vi "Bildunterschrifft.vi"(11 "Bildunterschrifft":string) -> (3 "Bildunterschrifft out":string)   [LabVIEW 2013]
panel:
  in  "OK Button":bool
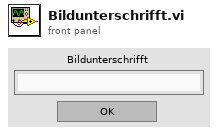
[diagram p1: front panel]
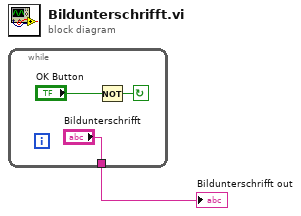
[diagram p0: block diagram]
diagram:
  n1 = while {
    tunnel: ["Bildunterschrifft"] -> w1
    stop <- w4 continue-if-true
    n2 = Not(x="OK Button") -> (.not. x?=w4:bool)
  }
  "Bildunterschrifft out" <- w1
